vi "Constants.vi"() -> ()   [LabVIEW 2016, in "UDP Sender Shared.lvlib"]
doc: "Use this Global VI to access the GUIDs assigned to the page resources of the Custom Device."
uses:
  UDP Sender Shared.lvlib
panel:
  in  "Tab Control":enum32{"GUIDS", "Constants", "Properties"}(tab)
  in  "UDP Sender":string="5f1fd38e-77fd-4c66-9fb4-50cec96d8a0f"
  in  "Destination Port":string="Destination Port"
  in  "Destination IP Address":string="Destination IP Address"
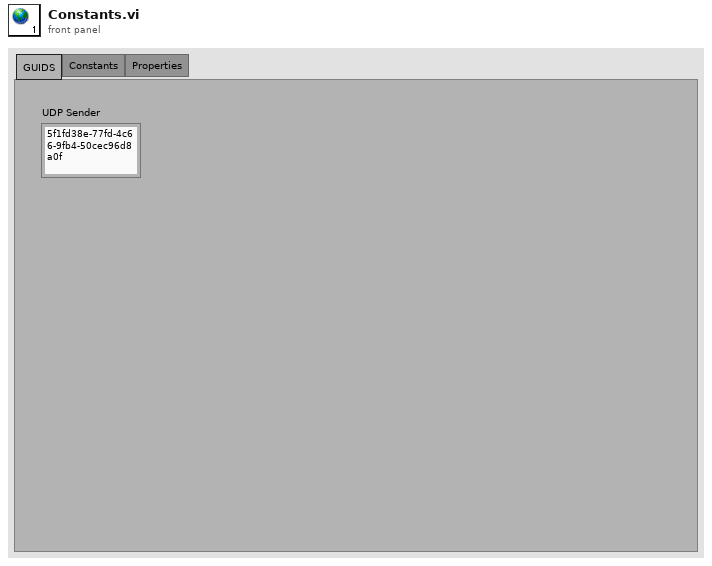
[diagram p1: front panel]
diagram:
